vi "系统 interface.vi"   [LabVIEW 2016, in "MB SLAVE.lvlib"]
uses:
  MB SLAVE.lvlib
types:
  T1 = typedef "系统交互.ctl" = cluster{"运行模式":enum16{"维护模式", "常规模式", "应急模式", "质控模式", "性能测试"}, "运行间隔":i16, "流程运行中":bool, "自动运行启动参数":T2, "SYSTEM Interface.总磷总氮类型":enum16{"单模块", "总磷总氮二合一模块", "氨氮总磷二合一模块"}, "多参数运行间隔":i16, "配水时间":dbl, "沉淀时间":dbl, "清洗时间":dbl, "关键参数改变":bool, "温度告警":bool, "湿度告警":bool, "烟感告警":bool, "水浸告警":bool, "开门告警":bool, "SystemTask":enum16{"停机", "待机", "调试", "水样采集", "沉沙", "进样", "仪表测试分析", "反吹", "清洗", "除藻"}, "PumpState":enum16{"--", "只用泵1", "只用泵2", "双泵交替"}, "除藻选择":enum16{"不开除藻", "开除藻"}, "报警信息":enum16{"无报警", "断电报警", "采样管理欠压（源水泵故障）", "进样管路欠压（进样泵/增加泵故障）"}, "软件升级":bool, "固件升级":enum16{"无", "CODMn", "氨氮", "总磷", "总氮", "CODCr"}, "数据传输软件升级":bool, "数采仪软件版本":string}
  T2 = typedef "启动参数.ctl" = cluster{"氨氮":bool, "总磷":bool, "总氮":bool, "多参数":bool, "CODmn":bool, "CODCr":bool, "氟化物":bool, "超标留样":bool, "重金属":bool, "挥发酚":bool}
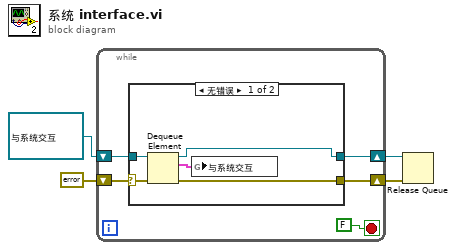
[diagram p0: block diagram]
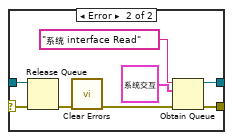
[diagram p2: hidden frame]
diagram:
  n1 = while {
    shift-right: [w9] -> w2
    shift-left: errorcluster {"status"=TRUE, "code"=0, "source"=""} ("error out") -> [w8]
    shift-right: [w6] -> w3
    shift-left: refnum<queue> refnum ("queue out") -> [w5]
    stop <- FALSE stop-if-true
    n2 = case shown="无错误" w8 {
      selector: w8 -> [w13 w20]
      tunnel: [w11 w21] -> w9
      tunnel: [w12 w16] -> w6
      tunnel: w5 -> [w14 w19]
      frame No Error {
        n3 = Dequeue Element(queue=w14, error in (no error)=w13) -> (queue out=w12:refnum<queue>, element=w10:T1, error out=w11:errorcluster)  [unwired: 1 in, 1 out]
        n4 = global write "modbus slave全局.vi" "与系统交互"(w10) -> ()
      }
      frame Error {
        n5 = Release Queue(queue=w19, error in (no error)=w20) -> (error out=w18:errorcluster)  [unwired: 1 in, 2 out]
        n6 = call <vilib>:"Clear Errors.vi"("error in (no error)"=w18) -> ("error out"=w17:errorcluster)  [unwired: 5 in, 1 out]
        n7 = Obtain Queue(name (unnamed)="系统 interface Read" ("写入方名称"), element data type=T1 {"运行模式"=enum."维护模式", "运行间隔"=4, "流程运行中"=FALSE, "自动运行启动参数"={"氨氮"=FALSE, "总磷"=FALSE, "总氮"=FALSE, "多参数"=FALSE, "CODmn"=FALSE, "CODCr"=FALSE, "氟化物"=FALSE, "超标留样"=FALSE, "重金属"=FALSE, "挥发酚"=FALSE}, "SYSTEM Interface.总磷总氮类型"=enum."单模块", "多参数运行间隔"=4, "配水时间"=0.0, "沉淀时间"=0.0, "清洗时间"=0.0, "关键参数改变"=FALSE, "温度告警"=FALSE, "湿度告警"=FALSE, "烟感告警"=FALSE, "水浸告警"=FALSE, "开门告警"=FALSE, "SystemTask"=enum."停机", "PumpState"=enum."--", "除藻选择"=enum."不开除藻", "报警信息"=enum."无报警", "软件升级"=FALSE, "固件升级"=enum."无", "数据传输软件升级"=FALSE, "数采仪软件版本"=""} ("与系统交互"), error in (no error)=w17) -> (queue out=w16:refnum<queue>, error out=w21:errorcluster)  [unwired: 2 in, 1 out]
      }
    }
  }
  n8 = Release Queue(queue=w3, error in (no error)=w2) -> ()  [unwired: 1 in, 3 out]
